vi "Ejercicio_20_customize.vi"() -> ()   [LabVIEW 2020]
panel:
  in  "Knob":dbl(knob) scale=0.0..10.0
  out "Slide":dbl(slide) scale=0.0..10.0
  out "Boolean 2":bool
  in  "Boolean":bool
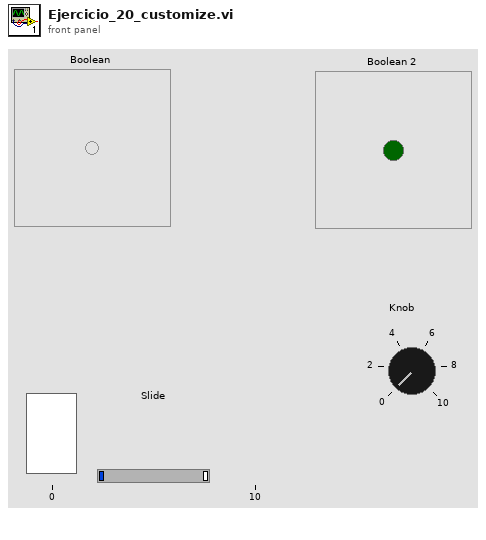
[diagram p1: front panel]
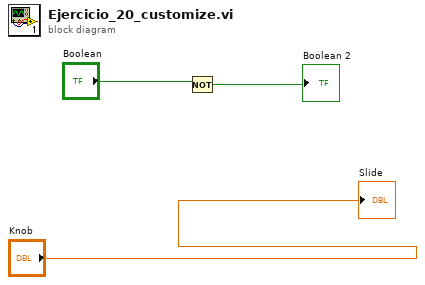
[diagram p0: block diagram]
diagram:
  n1 = Not(x="Boolean") -> (.not. x?=→"Boolean 2":bool)
  "Slide" <- "Knob"
